vi "Digital Filter.vi"(10 "Tics to Filter":fxp<+,11,11>, 11 "Input Signal":bool) -> (3 "Output Filtered Signal":bool)   [LabVIEW 2014]
doc: "This VI filters out digital glitches from Input Signal that are shorter than Tics to Filter. Tics to Filter specifies the time in multiple of FPGA tics inside a single cycle timed loop (normally 25 ns per tic).\nTics to filter set to 0 means filter disabled."
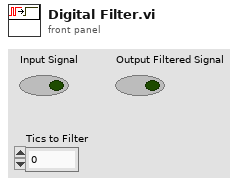
[diagram p1: front panel]
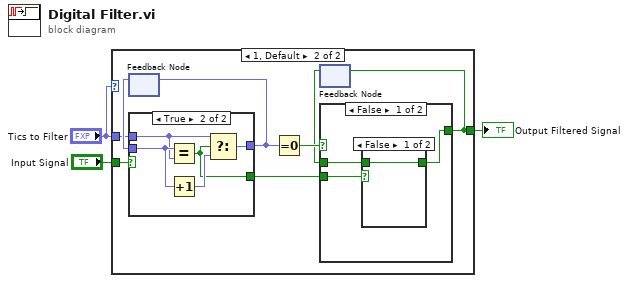
[diagram p0: block diagram]
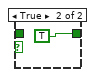
[diagram p3: hidden frame]
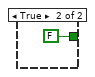
[diagram p4: hidden frame]
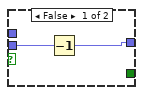
[diagram p5: hidden frame]
diagram:
  n1 = case shown="1, Default" "Tics to Filter" {
    tunnel: "Input Signal" -> [w4 w11]
    tunnel: "Tics to Filter" -> [_ w10]
    tunnel: [w4 w5] -> w2
    frame 0 {
      # "0 means filter disabled"
    }
    frame 1, Default {
      n2 = feedback #1() -> (w12:fxp<+,11,11>)  [unwired: 1 in]
      n3 = case shown="True" w11 {
        tunnel: [w19 w22] -> w9
        tunnel: w12 -> [w20 w25]
        tunnel: w10 -> [_ w23]
        tunnel: [_ w21] -> w6
        frame False {
          n4 = Decrement(x=w20) -> (x-1=w19:fxp<+,11,11>)
        }
        frame True {
          n5 = Equal?(x=w25, y=w23) -> (x = y?=w21:bool)
          n6 = Increment(x=w25) -> (x+1=w24:fxp<+,11,11>)
          n7 = Select(t=w23, s=w21, f=w24) -> (s? t:f=w22:fxp<+,11,11>)
        }
      }
      n8 = feedback-in #1(w9) -> ()
      n9 = Equal To 0?(x=w9) -> (x = 0?=w8:bool)
      n10 = feedback #2() -> (w7:bool)  [unwired: 1 in]
      n11 = case shown="False" w8 {
        tunnel: w7 -> [w13 _]
        tunnel: [w14 FALSE] -> w5
        tunnel: w6 -> [w15 _]
        frame False {
          n12 = case shown="False" w15 {
            tunnel: [w16 TRUE] -> w14
            tunnel: w13 -> [w16 _]
            frame False {
            }
            frame True {
            }
          }
        }
        frame True {
        }
      }
      n13 = feedback-in #2(w5) -> ()
    }
  }
  "Output Filtered Signal" <- w2
